vi "Autonomous Independent.vi"() -> ()   [LabVIEW 2017]
doc: "This VI is called when autonomous begins, and will automatically be terminated when autonomous ends. You can carry out timed or sensor driven robot movement independently without needing to return to the caller."
uses:
  <vilib>/Rock Robotics/WPI/ThirdParty/Phoenix-LabVIEW/Motor Controller/Controls/CTRE_Phoenix_MotorControl_ControlMode.ctl
  <vilib>/Rock Robotics/WPI/ThirdParty/Phoenix-LabVIEW/Pigeon IMU/CTRE_PigeonIMU_TareType.ctl
  Robot Global Data.vi
  <vilib>/Rock Robotics/Network Tables/NT Read Number.vi
panel:
  in  "Kp 4":dbl=0.015
  in  "Speed Dr str 4":dbl=1.0
  out "dis 3":i32
  out "Right Pos 2":i32
  in  "Kp 3":dbl=0.012
  in  "Speed Dr str 3":dbl=-0.5
  in  "Kp":dbl=0.015
  in  "Speed Dr str":dbl=1.0
  out "dis 2":i32
  out "Right Pos":i32
  in  "Kp 8":dbl=0.015
  in  "Speed Dr str 8":dbl=-1.0
  out "dis 7":i32
  out "Right Pos 6":i32
  in  "Kp 7":dbl=0.015
  in  "Speed Dr str 7":dbl=-1.0
  out "dis 6":i32
  out "Right Pos 5":i32
  in  "Kp 6":dbl=0.015
  in  "Speed Dr str 6":dbl=1.0
  out "dis 5":i32
  out "Right Pos 4":i32
  in  "Kp 5":dbl=0.015
  in  "Speed Dr str 5":dbl=-0.75
  in  "Kp 2":dbl=0.015
  in  "Speed Dr str 2":dbl=1.0
  out "dis 4":i32
  out "Right Pos 3":i32
  in  "First move (ms) 2":i32=60
  in  "First move Right 2":dbl=-0.75
  in  "First Move Left 2":dbl=-0.75
  # "Be sure to right-click and choose Data Operations>>Make Current Value default if you want to save the array values with the VI"
  # "115in from wall to swicth"
  # "SWITCH"
  # "SCALE"
  # "Correct"
  # "STRAIGHT SWITCH"
  # "-220"
  # "L"
  # "Staright auto"
  # ".117"
  # ".0041"
  # "=========================================================="
  # "Not correct"
  # "Get cube other side"
  # "R"
  # "other side"
  # "put 2nd cube in scale"
  # "find cube"
  # "waypt drive"
  # "Switch(new) Left"
  # "Switch(new) Right"
types:
  T1 = enum16{"FollowerType_PercentOutput", "FollowerType_AuxOutput1"}
  T2 = typedef "CTRE_PigeonIMU_TareType.ctl" = u8
  T3 = typedef "CTRE_Phoenix_MotorControl_ControlMode.ctl" = u16
  T4 = typedef "WPI_MotorControlDeviceRef.ctl" = cluster{"DeviceStatus":errorcluster, "Type":T5, "PWM":cluster{"PWM Channel":T6, "DeadBand":T7}, "CAN":cluster{"Device Number":u8, "SetOutput VI Ref":variant, "GetOutput VI Ref":variant, "Enable VI Ref":variant, "Disable VI Ref":variant, "Data":variant}, "Invert":bool, "DIO PWM":cluster{"PWM \"Enable\" Channel":T6, "DIOChannel":T8, "PWM Rate":dbl}}
  T5 = typedef "WPI_MotorControlType.ctl" = enum16{"PWM", "CAN", "DIO PWM"}
  T6 = typedef "FPGA_DIOPWMChannel.ctl" = enum8{"PWM 0", "PWM 1", "PWM 2", "PWM 3", "PWM 4", "PWM 5", "PWM 6", "PWM 7", "PWM 8", "PWM 9", "PWM MXP 0", "PWM MXP 1", "PWM MXP 2", "PWM MXP 3", "PWM MXP 4", "PWM MXP 5", "PWM MXP 6", "PWM MXP 7", "PWM MXP 8", "PWM MXP 9", "Invalid"}
  T7 = typedef "WPI_PWMDeadband.ctl" = cluster{"Name":string, "maxPositivePwm":i32, "minPositivePwm":i32, "centerPwm":i32, "maxNegativePwm":i32, "minNegativePwm":i32, "angularRange":u16}
  T8 = typedef "FPGA_DIOChannel.ctl" = enum8{"DIO 0", "DIO 1", "DIO 2", "DIO 3", "DIO 4", "DIO 5", "DIO 6", "DIO 7", "DIO 8", "DIO 9", "DIO MXP 0", "DIO MXP 1", "DIO MXP 2", "DIO MXP 3", "DIO MXP 4", "DIO MXP 5", "DIO MXP 6", "DIO MXP 7", "DIO MXP 8", "DIO MXP 9", "DIO MXP 10", "DIO MXP 11", "DIO MXP 12", "DIO MXP 13", "DIO MXP 14", "DIO MXP 15", "SPI Port CS1", "SPI Port CS2", "SPI Port CS3", "SPI Port MISO", "SPI Port MOSI", "Invalid"}
  T9 = typedef "CTRE_PigeonIMU_DeviceRef.ctl" = cluster{"DeviceStatus":errorcluster, "Device Number":u8, "Type":T10, "Device ID":u32, "Handle":u64, "UsageFrame":u32, "Library Path":path}
  T10 = typedef "CTRE_PigeonIMU_ConnectionType.ctl" = u32
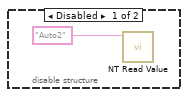
[diagram p2: hidden frame]
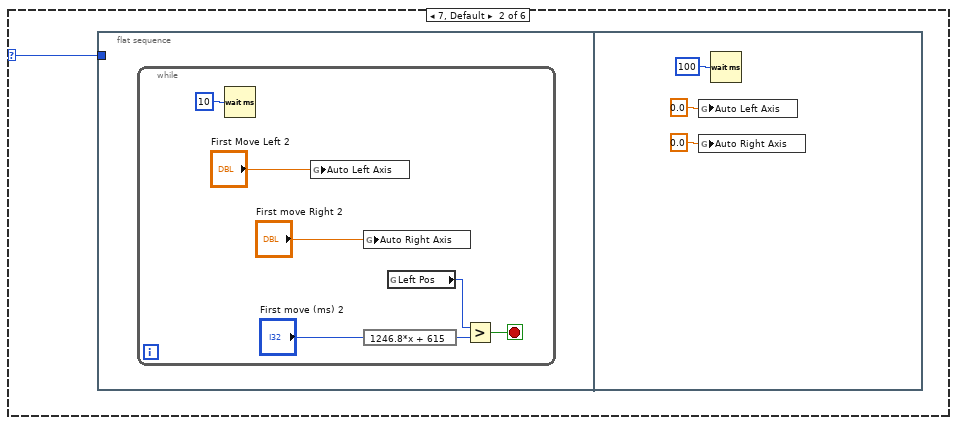
[diagram p3: hidden frame]
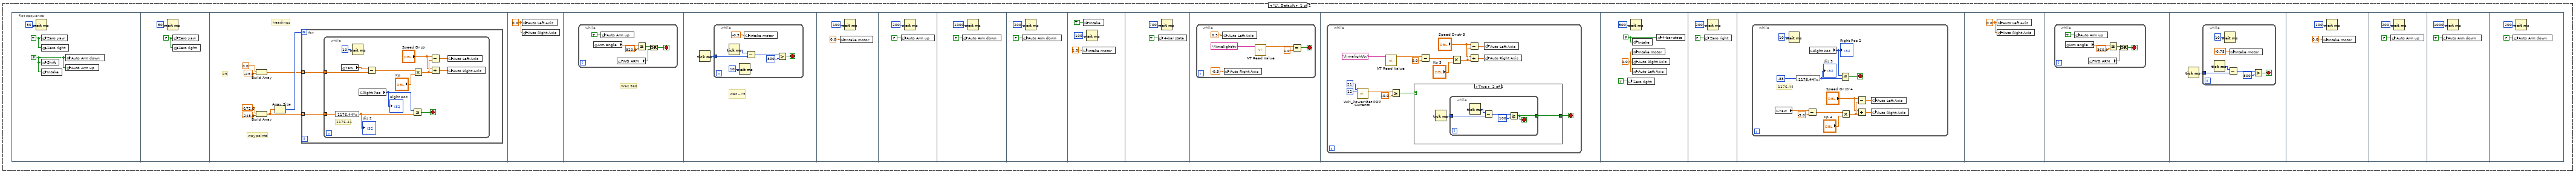
[diagram p5: hidden frame]
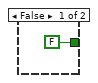
[diagram p6: hidden frame]
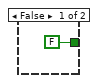
[diagram p7: hidden frame]
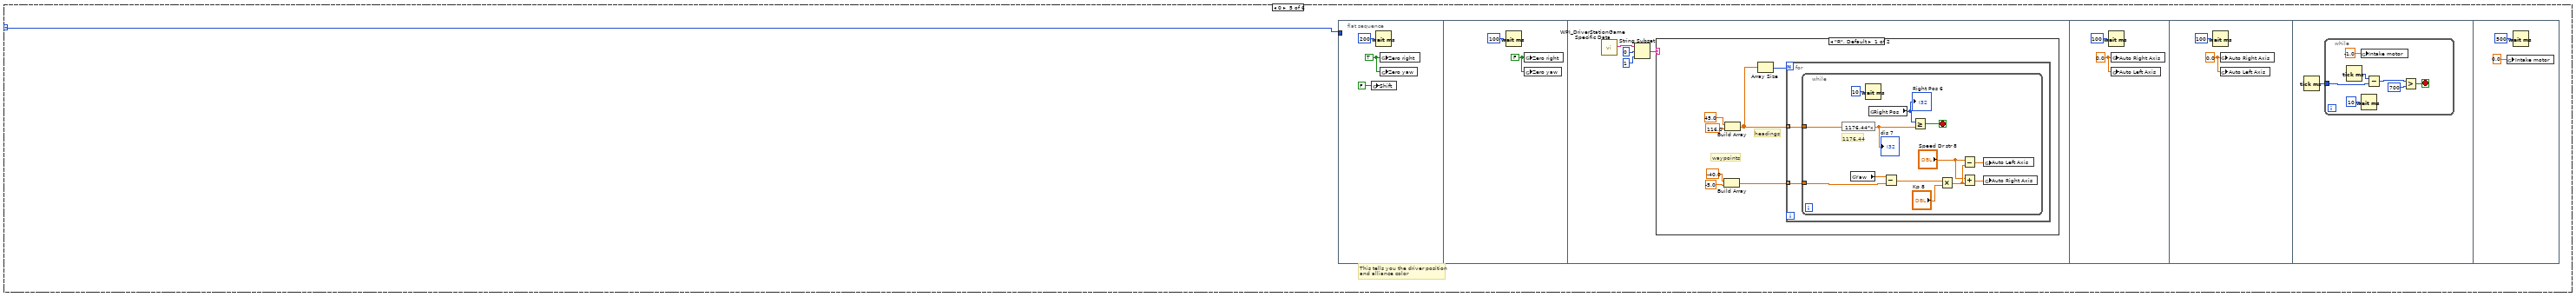
[diagram p9: hidden frame]
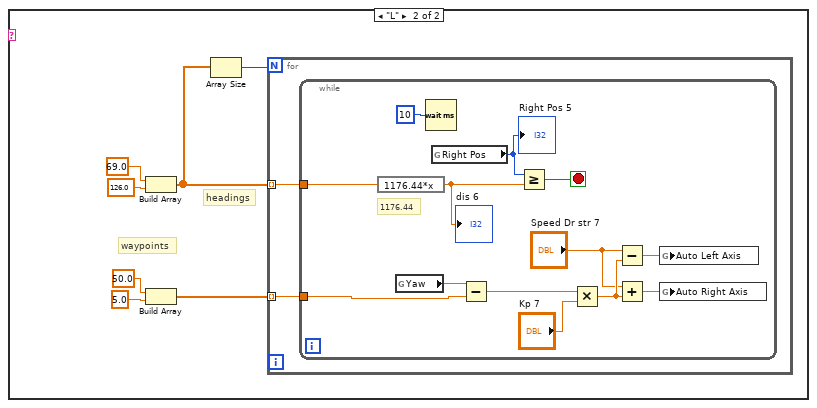
[diagram p10: hidden frame]
diagram:
  (unwired) "This function is run in parallel when the autonomous period begins. It will be terminated automatically when the period ends.\n\nNote that all Driver Station inputs are automatically latched and will not change once auto begins."
  # "Use time and/or sensors to control how the robot drives."
  # "Every 20ms, report that we are running autonomous\ncode. Loop will abort the same time as the VI."
  n1 = disable-structure shown="Enabled" {
    frame Disabled {
      n2 = call-poly <vilib>:"NT Read Value.vi"("Name"="Auto2") -> ()  [unwired: 9 in, 2 out]
    }
    frame Enabled {
    }
  }
  n3 = while {
    stop <- FALSE stop-if-true
    n4 = call <vilib>:"WPI_DriverStationReport Robot Code State.vi"("Autonomous"=TRUE) -> ()  [unwired: 10 in, 1 out]
    n5 = Wait (ms)(milliseconds to wait=u32 20) -> ()  [unwired: 1 out]
  }
  n6 = case shown="9" 9 {
    selector: 9 -> [_ w42 _ _ w336 _]
    frame 9 {
      w16 = T2 0 items=["SetValue"=0, "AddOffset"=1, "MatchCompass"=2, "SetOffset"=255] ("TareType (SetValue)")
      w6 = 0 ("New Sensor Position")
      w28 = 0.0 ("Output")
      w29 = T3 10 items=["PercentOutput"=0, "Position"=1, "Velocity"=2, "Current"=3, "Follower"=5, "MotionProfile"=6, "MotionMagic"=7, "MotionMagicArc"=8, "MotionProfileArc"=10, "Disabled"=15] ("Control Mode")
      w31 = T3 10 items=["PercentOutput"=0, "Position"=1, "Velocity"=2, "Current"=3, "Follower"=5, "MotionProfile"=6, "MotionMagic"=7, "MotionMagicArc"=8, "MotionProfileArc"=10, "Disabled"=15] ("Control Mode")
      n7 = call <vilib>:"CTRE_Phoenix_MotorControl_RefNumRegistryGet.vi"("refnum name"="Left encode") -> ("error out"=w26:errorcluster, "PhoenixMotorControlDevRef"=w24:T4)  [unwired: 9 in]
      n8 = call <vilib>:"CTRE_Phoenix_MotorControl_RefNumRegistryGet.vi"("refnum name"="Right encode") -> ("error out"=w27:errorcluster, "PhoenixMotorControlDevRef"=w23:T4)  [unwired: 9 in]
      n9 = call <vilib>:"CTRE_Phoenix_MotorControl_Set.vi"("error in (no error)"=w26, "Output"=w28, "Control Mode"=w29, "PhoenixMotorControlDevRef"=w24) -> ("error out"=w11:errorcluster, "PhoenixMotorControlDevRef"=w12:T4)  [unwired: 6 in]
      n10 = call <vilib>:"CTRE_Phoenix_MotorControl_Set.vi"("error in (no error)"=w27, "Output"=w28, "Control Mode"=w29, "PhoenixMotorControlDevRef"=w23) -> ("error out"=w7:errorcluster, "PhoenixMotorControlDevRef"=w10:T4)  [unwired: 6 in]
      n11 = call <vilib>:"CTRE_PigeonIMU_RefNumRegistryGet.vi"("refnum name"="imu") -> ("error out"=w14:errorcluster, "PigeonIMUDevRef"=w19:T9)  [unwired: 9 in]
      n12 = call <vilib>:"CTRE_Phoenix_MotorControl_SetQuadraturePosition_Enhanced.vi"("error in (no error)"=w11, "New Position"=w6, "PhoenixMotorControlDevRef"=w12) -> ("PhoenixMotorControlDevRef"=w13:T4)  [unwired: 7 in, 1 out]
      n13 = call <vilib>:"CTRE_Phoenix_MotorControl_SetQuadraturePosition_Enhanced.vi"("error in (no error)"=w7, "New Position"=w6, "PhoenixMotorControlDevRef"=w10) -> ("error out"=w8:errorcluster, "PhoenixMotorControlDevRef"=w9:T4)  [unwired: 7 in]
      n14 = call <vilib>:"CTRE_PigeonIMU_SetYaw.vi"("error in (no error)"=w14, "TareType (SetValue)"=w16, "Value"=0.0, "PigeonIMUDevRef"=w19) -> ()  [unwired: 6 in, 2 out]
      n15 = call <vilib>:"CTRE_Phoenix_MotorControl_ClearMotionProfileTrajectories.vi"("PhoenixMotorControlDevRef"=w9, "error in"=w8) -> ("PhoenixMotorControlDevRef"=w22:T4)  [unwired: 12 in, 1 out]
      n16 = call "Load Motion Profile.vi"("file path (dialog if empty)"=path "/home/lvuser/trajectories/right_cross.csv", "Right_Talon"=w22) -> ()  [unwired: 10 in]
      n17 = while {
        tunnel: [w39] -> w21
        tunnel: w13 -> [w39]
        tunnel: [w38] -> w15
        tunnel: w22 -> [w38]
        stop <- w41 stop-if-true
        n18 = global read "Robot Global Data.vi" "MP Cursor"() -> (w37:i32)
        n19 = Greater Or Equal?(x=w37, y=5) -> (x >= y?=w41:bool)
      }
      n20 = call <vilib>:"CTRE_Phoenix_MotorControl_Set.vi"("Output"=1.0, "Control Mode"=w31, "PhoenixMotorControlDevRef"=w15) -> ()  [unwired: 7 in, 2 out]
      n21 = call <vilib>:"CTRE_Phoenix_MotorControl_Follow.vi"("FollowerType"=T1."FollowerType_AuxOutput1", "Master Controller to Follow"=w15, "PhoenixMotorControlDevRef"=w21) -> ()  [unwired: 7 in, 2 out]
      n22 = while {
        tunnel: w15 -> [w36]
        stop <- FALSE stop-if-true
        n23 = call <vilib>:"CTRE_Phoenix_MotorControl_ProcessMotionProfileBuffer.vi"("PhoenixMotorControlDevRef"=w36) -> ()  [unwired: 13 in, 2 out]
        n24 = Wait (ms)(milliseconds to wait=u32 5) -> ()  [unwired: 1 out]
      }
    }
    frame 7, Default {
      n25 = flat-sequence {
        tunnel: w42 -> [_]
        frame #0 {
          n26 = while {
            stop <- w49 stop-if-true
            n27 = Wait (ms)(milliseconds to wait=u32 10) -> ()  [unwired: 1 out]
            n28 = global write "Robot Global Data.vi" "Auto Left Axis"("First Move Left 2") -> ()
            n29 = global write "Robot Global Data.vi" "Auto Right Axis"("First move Right 2") -> ()
            n30 = expression code="1246.8*x + 615"("First move (ms) 2") -> (w44:i32)
            n31 = global read "Robot Global Data.vi" "Left Pos"() -> (w43:i32)
            n32 = Greater?(x=w43, y=w44) -> (0:w49:bool)
          }
        }
        frame #1 {
          n33 = global write "Robot Global Data.vi" "Auto Left Axis"(0.0 ("Auto Left Axis")) -> ()
          n34 = global write "Robot Global Data.vi" "Auto Right Axis"(0.0 ("Auto Left Axis")) -> ()
          n35 = Wait (ms)(milliseconds to wait=u32 100) -> ()  [unwired: 1 out]
        }
      }
    }
    frame 3 {
      n36 = call <vilib>:"WPI_DriverStationGame Specific Data.vi"() -> ("Game Specific Data"=w56:string)  [unwired: 11 in]
      n37 = String Subset(string=w56, offset (0)=1, length (rest)=1 ("length (rest)")) -> (substring=w53:string)
      n38 = case shown="\"R\"" w53 {
        frame "L", Default {
          n39 = flat-sequence {
            frame #0 {
              w57 = FALSE
              w58 = TRUE ("Zero right")
              n40 = Wait (ms)(milliseconds to wait=u32 50) -> ()  [unwired: 1 out]
              n41 = global write "Robot Global Data.vi" "Zero yaw"(w58) -> ()
              n42 = global write "Robot Global Data.vi" "Zero right"(w58) -> ()
              n43 = global write "Robot Global Data.vi" "Shift"(w57) -> ()
              n44 = global write "Robot Global Data.vi" "Intake"(w57) -> ()
              n45 = global write "Robot Global Data.vi" "Auto Arm down"(w57) -> ()
              n46 = global write "Robot Global Data.vi" "Auto Arm up"(w57) -> ()
            }
            frame #1 {
              w60 = FALSE ("Zero right")
              n47 = Wait (ms)(milliseconds to wait=u32 50) -> ()  [unwired: 1 out]
              n48 = global write "Robot Global Data.vi" "Zero yaw"(w60) -> ()
              n49 = global write "Robot Global Data.vi" "Zero right"(w60) -> ()
            }
            frame #2 {
              # "25"
              # "waypoints"
              # "headings"
              n50 = Build Array(0.0 ("element"), -23.0 ("element")) -> (w62:dbl[])
              n51 = Build Array(-172.0 ("element"), -248.0 ("element")) -> (w63:dbl[])
              n52 = Array Size(array=w63) -> (size(s)=w68:i32)
              n53 = for {
                N: w68 -> [_]
                tunnel: w63 -> [w70] mode=indexing
                tunnel: w62 -> [w69] mode=indexing
                n54 = while {
                  tunnel: w70 -> [w75]
                  tunnel: w69 -> [w71]
                  stop <- w80 stop-if-true
                  # "1176.44"
                  n55 = expression code="1176.44*x"(w75) -> (w76:dbl)
                  "dis 2" <- w76
                  n56 = global read "Robot Global Data.vi" "Yaw"() -> (w72:dbl)
                  n57 = Wait (ms)(milliseconds to wait=u32 10) -> ()  [unwired: 1 out]
                  n58 = global read "Robot Global Data.vi" "Right Pos"() -> (w73:i32)
                  "Right Pos" <- w73
                  n59 = Subtract(x=w72, y=w71) -> (x-y=w74:dbl)
                  n60 = Less Or Equal?(x=w73, y=w76) -> (x <= y?=w80:bool)
                  n61 = Multiply(x=w74, y="Kp") -> (x*y=w79:dbl)
                  n62 = Subtract(x="Speed Dr str", y=w79) -> (x-y=w82:dbl)
                  n63 = Add(x="Speed Dr str", y=w79) -> (x+y=w81:dbl)
                  n64 = global write "Robot Global Data.vi" "Auto Left Axis"(w82) -> ()
                  n65 = global write "Robot Global Data.vi" "Auto Right Axis"(w81) -> ()
                }
              }
            }
            frame #3 {
              w84 = 0.0
              n66 = global write "Robot Global Data.vi" "Auto Left Axis"(w84) -> ()
              n67 = global write "Robot Global Data.vi" "Auto Right Axis"(w84) -> ()
            }
            frame #4 {
              # "Was 360"
              n68 = while {
                stop <- w85 stop-if-true
                n69 = global read "Robot Global Data.vi" "Arm angle"() -> (w89:dbl)
                n70 = global write "Robot Global Data.vi" "Auto Arm up"(TRUE) -> ()
                n71 = global read "Robot Global Data.vi" "FWD ARM"() -> (w86:bool)
                n72 = Greater Or Equal?(x=w89, y=320.0) -> (x >= y?=w87:bool)
                n73 = Or(x=w87, y=w86) -> (x .or. y?=w85:bool)
              }
            }
            frame #5 {
              # "was -.75"
              n74 = Tick Count (ms)() -> (millisecond timer value=w91:u32)
              n75 = while {
                tunnel: w91 -> [w96]
                stop <- w93 stop-if-true
                n76 = Tick Count (ms)() -> (millisecond timer value=w97:u32)
                n77 = Wait (ms)(milliseconds to wait=u32 10) -> ()  [unwired: 1 out]
                n78 = global write "Robot Global Data.vi" "Intake motor"(-0.5 ("Intake motor")) -> ()
                n79 = Subtract(x=w97, y=w96) -> (x-y=w95:u32)
                n80 = Greater?(x=w95, y=u32 800) -> (0:w93:bool)
              }
            }
            frame #6 {
              n81 = global write "Robot Global Data.vi" "Intake motor"(0.0 ("Intake motor")) -> ()
              n82 = Wait (ms)(milliseconds to wait=u32 100) -> ()  [unwired: 1 out]
            }
            frame #7 {
              n83 = global write "Robot Global Data.vi" "Auto Arm up"(FALSE) -> ()
              n84 = Wait (ms)(milliseconds to wait=u32 200) -> ()  [unwired: 1 out]
            }
            frame #8 {
              n85 = global write "Robot Global Data.vi" "Auto Arm down"(TRUE) -> ()
              n86 = Wait (ms)(milliseconds to wait=u32 1000) -> ()  [unwired: 1 out]
            }
            frame #9 {
              n87 = global write "Robot Global Data.vi" "Auto Arm down"(FALSE) -> ()
              n88 = Wait (ms)(milliseconds to wait=u32 200) -> ()  [unwired: 1 out]
            }
            frame #10 {
              n89 = global write "Robot Global Data.vi" "Intake motor"(1.0 ("Intake motor")) -> ()
              n90 = global write "Robot Global Data.vi" "Intake"(TRUE ("Intake")) -> ()
              n91 = Wait (ms)(milliseconds to wait=u32 100) -> ()  [unwired: 1 out]
            }
            frame #11 {
              n92 = global write "Robot Global Data.vi" "4-bar state"(TRUE ("4-bar state")) -> ()
              n93 = Wait (ms)(milliseconds to wait=u32 700) -> ()  [unwired: 1 out]
            }
            frame #12 {
              n94 = while {
                stop <- w112 stop-if-true
                n95 = global write "Robot Global Data.vi" "Auto Left Axis"(0.5 ("Auto Left Axis")) -> ()
                n96 = global write "Robot Global Data.vi" "Auto Right Axis"(-0.5 ("Auto Right Axis")) -> ()
                n97 = call-poly <vilib>:"NT Read Value.vi"("Name"="/limelight/tv") -> ("Numeric"=w114:dbl)  [unwired: 9 in, 1 out]
                n98 = Equal?(x=w114, y=1.0) -> (x = y?=w112:bool)
              }
            }
            frame #13 {
              n99 = while {
                stop <- w132 stop-if-true
                n100 = call <vilib>:"WPI_Power Get PDP Currents.vi"("Power Distribution Panel (0)"=u8 21, "PDP Channel"=12) -> ("current (A)"=w127:dbl)  [unwired: 11 in, 2 out]
                n101 = call-poly <vilib>:"NT Read Value.vi"("Name"="/limelight/tx") -> ("Numeric"=w119:dbl)  [unwired: 9 in, 1 out]
                n102 = Greater Or Equal?(x=w127, y=40.0 ("x")) -> (x >= y?=w129:bool)
                n103 = case shown="True" w129 {
                  tunnel: [FALSE w134] -> w132
                  frame False {
                  }
                  frame True {
                    n104 = Tick Count (ms)() -> (millisecond timer value=w135:u32)
                    n105 = while {
                      tunnel: w135 -> [w139]
                      tunnel: [w136] -> w134
                      stop <- w136 stop-if-true
                      n106 = Tick Count (ms)() -> (millisecond timer value=w140:u32)
                      n107 = Subtract(x=w140, y=w139) -> (x-y=w138:u32)
                      n108 = Greater Or Equal?(x=w138, y=u32 100) -> (x >= y?=w136:bool)
                    }
                  }
                }
                n109 = Subtract(x=w119, y=0.0) -> (x-y=w121:dbl)
                n110 = Multiply(x=w121, y="Kp 3") -> (x*y=w123:dbl)
                n111 = Subtract(x="Speed Dr str 3", y=w123) -> (x-y=w125:dbl)
                n112 = Add(x="Speed Dr str 3", y=w123) -> (x+y=w124:dbl)
                n113 = global write "Robot Global Data.vi" "Auto Left Axis"(w125) -> ()
                n114 = global write "Robot Global Data.vi" "Auto Right Axis"(w124) -> ()
              }
            }
            frame #14 {
              w141 = FALSE ("4-bar state")
              w144 = 0.0 ("Intake motor")
              n115 = global write "Robot Global Data.vi" "Zero right"(TRUE) -> ()
              n116 = Wait (ms)(milliseconds to wait=u32 500) -> ()  [unwired: 1 out]
              n117 = global write "Robot Global Data.vi" "Intake"(w141) -> ()
              n118 = global write "Robot Global Data.vi" "Intake motor"(w144) -> ()
              n119 = global write "Robot Global Data.vi" "Auto Right Axis"(w144) -> ()
              n120 = global write "Robot Global Data.vi" "Auto Left Axis"(w144) -> ()
              n121 = global write "Robot Global Data.vi" "4-bar state"(w141) -> ()
            }
            frame #15 {
              n122 = global write "Robot Global Data.vi" "Zero right"(FALSE) -> ()
              n123 = Wait (ms)(milliseconds to wait=u32 200) -> ()  [unwired: 1 out]
            }
            frame #16 {
              n124 = while {
                stop <- w156 stop-if-true
                # "1176.44"
                n125 = global read "Robot Global Data.vi" "Yaw"() -> (w150:dbl)
                n126 = Wait (ms)(milliseconds to wait=u32 10) -> ()  [unwired: 1 out]
                n127 = expression code="1176.44*x"(-35) -> (w152:i32)
                "dis 3" <- w152
                n128 = Subtract(x=w150, y=-5.0) -> (x-y=w151:dbl)
                n129 = global read "Robot Global Data.vi" "Right Pos"() -> (w149:i32)
                "Right Pos 2" <- w149
                n130 = Less Or Equal?(x=w149, y=w152) -> (x <= y?=w156:bool)
                n131 = Multiply(x=w151, y="Kp 4") -> (x*y=w155:dbl)
                n132 = Subtract(x="Speed Dr str 4", y=w155) -> (x-y=w158:dbl)
                n133 = Add(x="Speed Dr str 4", y=w155) -> (x+y=w157:dbl)
                n134 = global write "Robot Global Data.vi" "Auto Left Axis"(w158) -> ()
                n135 = global write "Robot Global Data.vi" "Auto Right Axis"(w157) -> ()
              }
            }
            frame #17 {
              w160 = 0.0
              n136 = global write "Robot Global Data.vi" "Auto Left Axis"(w160) -> ()
              n137 = global write "Robot Global Data.vi" "Auto Right Axis"(w160) -> ()
            }
            frame #18 {
              n138 = while {
                stop <- w161 stop-if-true
                n139 = global read "Robot Global Data.vi" "Arm angle"() -> (w165:dbl)
                n140 = global write "Robot Global Data.vi" "Auto Arm up"(TRUE) -> ()
                n141 = global read "Robot Global Data.vi" "FWD ARM"() -> (w162:bool)
                n142 = Greater Or Equal?(x=w165, y=360.0) -> (x >= y?=w163:bool)
                n143 = Or(x=w163, y=w162) -> (x .or. y?=w161:bool)
              }
            }
            frame #19 {
              n144 = Tick Count (ms)() -> (millisecond timer value=w167:u32)
              n145 = while {
                tunnel: w167 -> [w172]
                stop <- w169 stop-if-true
                n146 = Tick Count (ms)() -> (millisecond timer value=w173:u32)
                n147 = Wait (ms)(milliseconds to wait=u32 10) -> ()  [unwired: 1 out]
                n148 = Subtract(x=w173, y=w172) -> (x-y=w171:u32)
                n149 = global write "Robot Global Data.vi" "Intake motor"(-0.75 ("Intake motor")) -> ()
                n150 = Greater?(x=w171, y=u32 800) -> (0:w169:bool)
              }
            }
            frame #20 {
              n151 = global write "Robot Global Data.vi" "Intake motor"(0.0 ("Intake motor")) -> ()
              n152 = Wait (ms)(milliseconds to wait=u32 100) -> ()  [unwired: 1 out]
            }
            frame #21 {
              n153 = global write "Robot Global Data.vi" "Auto Arm up"(FALSE) -> ()
              n154 = Wait (ms)(milliseconds to wait=u32 200) -> ()  [unwired: 1 out]
            }
            frame #22 {
              n155 = global write "Robot Global Data.vi" "Auto Arm down"(TRUE) -> ()
              n156 = Wait (ms)(milliseconds to wait=u32 1000) -> ()  [unwired: 1 out]
            }
            frame #23 {
              n157 = global write "Robot Global Data.vi" "Auto Arm down"(FALSE) -> ()
              n158 = Wait (ms)(milliseconds to wait=u32 200) -> ()  [unwired: 1 out]
            }
          }
        }
        frame "R" {
          # "other side"
          n159 = flat-sequence {
            frame #0 {
              w187 = TRUE ("4-bar state")
              n160 = global write "Robot Global Data.vi" "Auto Right Axis"(0.0 ("Auto Right Axis")) -> ()
              n161 = global write "Robot Global Data.vi" "Auto Left Axis"(0.0 ("Auto Left Axis")) -> ()
              n162 = global write "Robot Global Data.vi" "4-bar state"(FALSE ("4-bar state")) -> ()
              n163 = Wait (ms)(milliseconds to wait=u32 50) -> ()  [unwired: 1 out]
              n164 = global write "Robot Global Data.vi" "Zero right"(w187) -> ()
              n165 = global write "Robot Global Data.vi" "Zero yaw"(w187) -> ()
            }
            frame #1 {
              w189 = FALSE ("4-bar state")
              n166 = Wait (ms)(milliseconds to wait=u32 50) -> ()  [unwired: 1 out]
              n167 = global write "Robot Global Data.vi" "Zero right"(w189) -> ()
              n168 = global write "Robot Global Data.vi" "Zero yaw"(w189) -> ()
            }
            frame #2 {
              # "-237"
              # "-400"
              # "waypoints"
              # "headings"
              n169 = Build Array(-170.0 ("element"), -200.0 ("element"), -237.0 ("element"), -400.0 ("element")) -> (w195:dbl[])
              n170 = Array Size(array=w195) -> (size(s)=w200:i32)
              n171 = Build Array(0.0 ("element"), -30.0 ("element"), -90.0 ("element"), -90.0 ("element")) -> (w194:dbl[])
              n172 = for {
                N: w200 -> [_]
                tunnel: w195 -> [w202] mode=indexing
                tunnel: w194 -> [w201] mode=indexing
                n173 = while {
                  tunnel: w202 -> [w207]
                  tunnel: w201 -> [w203]
                  stop <- w212 stop-if-true
                  # "1176.44"
                  n174 = expression code="1176.44*x"(w207) -> (w208:dbl)
                  "dis 4" <- w208
                  n175 = global read "Robot Global Data.vi" "Yaw"() -> (w204:dbl)
                  n176 = Wait (ms)(milliseconds to wait=u32 10) -> ()  [unwired: 1 out]
                  n177 = global read "Robot Global Data.vi" "Right Pos"() -> (w205:i32)
                  "Right Pos 3" <- w205
                  n178 = Subtract(x=w204, y=w203) -> (x-y=w206:dbl)
                  n179 = Less Or Equal?(x=w205, y=w208) -> (x <= y?=w212:bool)
                  n180 = Multiply(x=w206, y="Kp 2") -> (x*y=w211:dbl)
                  n181 = Subtract(x="Speed Dr str 2", y=w211) -> (x-y=w214:dbl)
                  n182 = Add(x="Speed Dr str 2", y=w211) -> (x+y=w213:dbl)
                  n183 = global write "Robot Global Data.vi" "Auto Left Axis"(w214) -> ()
                  n184 = global write "Robot Global Data.vi" "Auto Right Axis"(w213) -> ()
                }
              }
            }
            frame #3 {
              w216 = 0.0
              n185 = global write "Robot Global Data.vi" "Auto Left Axis"(w216) -> ()
              n186 = global write "Robot Global Data.vi" "Auto Right Axis"(w216) -> ()
            }
            frame #4 {
              n187 = while {
                stop <- w218 stop-if-true
                n188 = global read "Robot Global Data.vi" "Yaw"() -> (w220:dbl)
                n189 = Wait (ms)(milliseconds to wait=u32 10) -> ()  [unwired: 1 out]
                n190 = global write "Robot Global Data.vi" "Auto Left Axis"(0.75) -> ()
                n191 = global write "Robot Global Data.vi" "Auto Right Axis"(-0.75) -> ()
                n192 = Greater Or Equal?(x=w220, y=-15.0) -> (x >= y?=w218:bool)
              }
            }
            frame #5 {
              w224 = 0.0
              n193 = Wait (ms)(milliseconds to wait=u32 20) -> ()  [unwired: 1 out]
              n194 = global write "Robot Global Data.vi" "Auto Left Axis"(w224) -> ()
              n195 = global write "Robot Global Data.vi" "Auto Right Axis"(w224) -> ()
            }
            frame #6 {
              n196 = global write "Robot Global Data.vi" "Zero right"(TRUE ("Zero right")) -> ()
              n197 = Wait (ms)(milliseconds to wait=u32 150) -> ()  [unwired: 1 out]
            }
            frame #7 {
              n198 = global write "Robot Global Data.vi" "Zero right"(FALSE ("Zero right")) -> ()
              n199 = Wait (ms)(milliseconds to wait=u32 50) -> ()  [unwired: 1 out]
            }
            frame #8 {
              n200 = while {
                stop <- w230 stop-if-true
                w234 = 1.0
                n201 = Wait (ms)(milliseconds to wait=u32 10) -> ()  [unwired: 1 out]
                n202 = global write "Robot Global Data.vi" "Auto Left Axis"(w234) -> ()
                n203 = global write "Robot Global Data.vi" "Auto Right Axis"(w234) -> ()
                n204 = global read "Robot Global Data.vi" "Right Pos"() -> (w233:i32)
                n205 = expression code="1176.44*x"(-12.0 ("element")) -> (w232:dbl)
                n206 = Less Or Equal?(x=w233, y=w232) -> (x <= y?=w230:bool)
              }
            }
            frame #9 {
              w236 = 0.0
              n207 = Wait (ms)(milliseconds to wait=u32 20) -> ()  [unwired: 1 out]
              n208 = global write "Robot Global Data.vi" "Auto Left Axis"(w236) -> ()
              n209 = global write "Robot Global Data.vi" "Auto Right Axis"(w236) -> ()
            }
            frame #10 {
              # "was 300"
              n210 = while {
                stop <- w237 stop-if-true
                n211 = global read "Robot Global Data.vi" "Arm angle"() -> (w241:dbl)
                n212 = global write "Robot Global Data.vi" "Auto Arm up"(TRUE) -> ()
                n213 = global read "Robot Global Data.vi" "FWD ARM"() -> (w238:bool)
                n214 = Greater Or Equal?(x=w241, y=290.0) -> (x >= y?=w239:bool)
                n215 = Or(x=w239, y=w238) -> (x .or. y?=w237:bool)
              }
            }
            frame #11 {
              # "was -.5"
              n216 = Tick Count (ms)() -> (millisecond timer value=w243:u32)
              n217 = while {
                tunnel: w243 -> [w248]
                stop <- w245 stop-if-true
                n218 = Tick Count (ms)() -> (millisecond timer value=w249:u32)
                n219 = Wait (ms)(milliseconds to wait=u32 10) -> ()  [unwired: 1 out]
                n220 = global write "Robot Global Data.vi" "Intake motor"(-0.5 ("Intake motor")) -> ()
                n221 = Subtract(x=w249, y=w248) -> (x-y=w247:u32)
                n222 = Greater?(x=w247, y=u32 500) -> (0:w245:bool)
              }
            }
            frame #12 {
              n223 = global write "Robot Global Data.vi" "Intake motor"(0.0 ("Intake motor")) -> ()
              n224 = Wait (ms)(milliseconds to wait=u32 50) -> ()  [unwired: 1 out]
            }
            frame #13 {
              n225 = global write "Robot Global Data.vi" "Auto Arm up"(FALSE) -> ()
              n226 = global write "Robot Global Data.vi" "Auto Arm down"(TRUE ("Auto Arm down")) -> ()
              n227 = Wait (ms)(milliseconds to wait=u32 1000) -> ()  [unwired: 1 out]
            }
            frame #14 {
              n228 = global write "Robot Global Data.vi" "Auto Arm down"(FALSE) -> ()
              n229 = Wait (ms)(milliseconds to wait=u32 50) -> ()  [unwired: 1 out]
            }
            frame #15 {
              n230 = global write "Robot Global Data.vi" "Intake motor"(1.0 ("Intake motor")) -> ()
              n231 = global write "Robot Global Data.vi" "Intake"(TRUE ("Intake")) -> ()
              n232 = Wait (ms)(milliseconds to wait=u32 50) -> ()  [unwired: 1 out]
            }
            frame #16 {
              n233 = global write "Robot Global Data.vi" "4-bar state"(TRUE ("4-bar state")) -> ()
              n234 = Wait (ms)(milliseconds to wait=u32 700) -> ()  [unwired: 1 out]
            }
            frame #17 {
              n235 = Tick Count (ms)() -> (millisecond timer value=w263:u32)
              n236 = while {
                tunnel: w263 -> [w267]
                stop <- w264 stop-if-true
                n237 = Tick Count (ms)() -> (millisecond timer value=w268:u32)
                n238 = global write "Robot Global Data.vi" "Auto Right Axis"(1.0) -> ()
                n239 = global write "Robot Global Data.vi" "Auto Left Axis"(-1.0) -> ()
                n240 = Subtract(x=w268, y=w267) -> (x-y=w266:u32)
                n241 = Greater Or Equal?(x=w266, y=u32 100) -> (x >= y?=w264:bool)
              }
            }
            frame #18 {
              n242 = while {
                stop <- w285 stop-if-true
                n243 = call <vilib>:"WPI_Power Get PDP Currents.vi"("Power Distribution Panel (0)"=u8 21, "PDP Channel"=12) -> ("current (A)"=w280:dbl)  [unwired: 11 in, 2 out]
                n244 = call-poly <vilib>:"NT Read Value.vi"("Name"="/limelight/tx") -> ("Numeric"=w272:dbl)  [unwired: 9 in, 1 out]
                n245 = Greater Or Equal?(x=w280, y=40.0 ("x")) -> (x >= y?=w282:bool)
                n246 = case shown="True" w282 {
                  tunnel: [FALSE w287] -> w285
                  frame False {
                  }
                  frame True {
                    n247 = Tick Count (ms)() -> (millisecond timer value=w288:u32)
                    n248 = while {
                      tunnel: w288 -> [w292]
                      tunnel: [w289] -> w287
                      stop <- w289 stop-if-true
                      n249 = Tick Count (ms)() -> (millisecond timer value=w293:u32)
                      n250 = Subtract(x=w293, y=w292) -> (x-y=w291:u32)
                      n251 = Greater Or Equal?(x=w291, y=u32 70) -> (x >= y?=w289:bool)
                    }
                  }
                }
                n252 = Subtract(x=w272, y=0.0) -> (x-y=w274:dbl)
                n253 = Multiply(x=w274, y="Kp 5") -> (x*y=w276:dbl)
                n254 = Subtract(x="Speed Dr str 5", y=w276) -> (x-y=w278:dbl)
                n255 = Add(x="Speed Dr str 5", y=w276) -> (x+y=w277:dbl)
                n256 = global write "Robot Global Data.vi" "Auto Left Axis"(w278) -> ()
                n257 = global write "Robot Global Data.vi" "Auto Right Axis"(w277) -> ()
              }
            }
            frame #19 {
              w294 = FALSE ("4-bar state")
              w297 = 0.0 ("Intake motor")
              n258 = global write "Robot Global Data.vi" "Zero right"(TRUE) -> ()
              n259 = Wait (ms)(milliseconds to wait=u32 150) -> ()  [unwired: 1 out]
              n260 = global write "Robot Global Data.vi" "Intake"(w294) -> ()
              n261 = global write "Robot Global Data.vi" "Intake motor"(w297) -> ()
              n262 = global write "Robot Global Data.vi" "Auto Right Axis"(w297) -> ()
              n263 = global write "Robot Global Data.vi" "Auto Left Axis"(w297) -> ()
              n264 = global write "Robot Global Data.vi" "4-bar state"(w294) -> ()
            }
            frame #20 {
              n265 = global write "Robot Global Data.vi" "Zero right"(FALSE) -> ()
              n266 = Wait (ms)(milliseconds to wait=u32 50) -> ()  [unwired: 1 out]
            }
            frame #21 {
              n267 = while {
                stop <- w309 stop-if-true
                # "1176.44"
                n268 = global read "Robot Global Data.vi" "Yaw"() -> (w303:dbl)
                n269 = Wait (ms)(milliseconds to wait=u32 10) -> ()  [unwired: 1 out]
                n270 = expression code="1176.44*x"(-20) -> (w305:i32)
                "dis 5" <- w305
                n271 = Subtract(x=w303, y=0.0) -> (x-y=w304:dbl)
                n272 = global read "Robot Global Data.vi" "Right Pos"() -> (w302:i32)
                "Right Pos 4" <- w302
                n273 = Less Or Equal?(x=w302, y=w305) -> (x <= y?=w309:bool)
                n274 = Multiply(x=w304, y="Kp 6") -> (x*y=w308:dbl)
                n275 = Subtract(x="Speed Dr str 6", y=w308) -> (x-y=w311:dbl)
                n276 = Add(x="Speed Dr str 6", y=w308) -> (x+y=w310:dbl)
                n277 = global write "Robot Global Data.vi" "Auto Left Axis"(w311) -> ()
                n278 = global write "Robot Global Data.vi" "Auto Right Axis"(w310) -> ()
              }
            }
            frame #22 {
              w313 = 0.0
              n279 = global write "Robot Global Data.vi" "Auto Left Axis"(w313) -> ()
              n280 = global write "Robot Global Data.vi" "Auto Right Axis"(w313) -> ()
            }
            frame #23 {
              n281 = while {
                stop <- w314 stop-if-true
                n282 = global read "Robot Global Data.vi" "Arm angle"() -> (w318:dbl)
                n283 = global write "Robot Global Data.vi" "Auto Arm up"(TRUE) -> ()
                n284 = global read "Robot Global Data.vi" "FWD ARM"() -> (w315:bool)
                n285 = Greater Or Equal?(x=w318, y=300.0) -> (x >= y?=w316:bool)
                n286 = Or(x=w316, y=w315) -> (x .or. y?=w314:bool)
              }
            }
            frame #24 {
              n287 = Tick Count (ms)() -> (millisecond timer value=w320:u32)
              n288 = while {
                tunnel: w320 -> [w325]
                stop <- w322 stop-if-true
                n289 = Tick Count (ms)() -> (millisecond timer value=w326:u32)
                n290 = Wait (ms)(milliseconds to wait=u32 10) -> ()  [unwired: 1 out]
                n291 = global write "Robot Global Data.vi" "Intake motor"(-0.3 ("Intake motor")) -> ()
                n292 = Subtract(x=w326, y=w325) -> (x-y=w324:u32)
                n293 = Greater?(x=w324, y=u32 800) -> (0:w322:bool)
              }
            }
            frame #25 {
              n294 = global write "Robot Global Data.vi" "Intake motor"(0.0 ("Intake motor")) -> ()
              n295 = Wait (ms)(milliseconds to wait=u32 50) -> ()  [unwired: 1 out]
            }
            frame #26 {
              n296 = global write "Robot Global Data.vi" "Auto Arm up"(FALSE) -> ()
              n297 = Wait (ms)(milliseconds to wait=u32 200) -> ()  [unwired: 1 out]
            }
            frame #27 {
              n298 = global write "Robot Global Data.vi" "Auto Arm down"(TRUE) -> ()
              n299 = Wait (ms)(milliseconds to wait=u32 1000) -> ()  [unwired: 1 out]
            }
            frame #28 {
              n300 = global write "Robot Global Data.vi" "Auto Arm down"(FALSE) -> ()
              n301 = Wait (ms)(milliseconds to wait=u32 50) -> ()  [unwired: 1 out]
            }
          }
        }
      }
    }
    frame 1 {
    }
    frame 0 {
      # "This tells you the driver position\nand alliance color"
      n302 = flat-sequence {
        tunnel: w336 -> [_]
        frame #0 {
          w338 = TRUE
          n303 = global write "Robot Global Data.vi" "Shift"(FALSE ("Shift")) -> ()
          n304 = Wait (ms)(milliseconds to wait=u32 200) -> ()  [unwired: 1 out]
          n305 = global write "Robot Global Data.vi" "Zero right"(w338) -> ()
          n306 = global write "Robot Global Data.vi" "Zero yaw"(w338) -> ()
        }
        frame #1 {
          w340 = FALSE
          n307 = Wait (ms)(milliseconds to wait=u32 100) -> ()  [unwired: 1 out]
          n308 = global write "Robot Global Data.vi" "Zero right"(w340) -> ()
          n309 = global write "Robot Global Data.vi" "Zero yaw"(w340) -> ()
        }
        frame #2 {
          n310 = call <vilib>:"WPI_DriverStationGame Specific Data.vi"() -> ("Game Specific Data"=w345:string)  [unwired: 11 in]
          n311 = String Subset(string=w345, offset (0)=0, length (rest)=1 ("length (rest)")) -> (substring=w342:string)
          n312 = case shown="\"R\", Default" w342 {
            frame "R", Default {
              # "waypoints"
              # "headings"
              n313 = Build Array(-40.0 ("element"), -5.0 ("element")) -> (w352:dbl[])
              n314 = Build Array(45.0 ("element"), 116.0 ("element")) -> (w351:dbl[])
              n315 = Array Size(array=w351) -> (size(s)=w350:i32)
              n316 = for {
                N: w350 -> [_]
                tunnel: w351 -> [w354] mode=indexing
                tunnel: w352 -> [w353] mode=indexing
                n317 = while {
                  tunnel: w354 -> [w359]
                  tunnel: w353 -> [w355]
                  stop <- w364 stop-if-true
                  # "1176.44"
                  n318 = expression code="1176.44*x"(w359) -> (w360:dbl)
                  "dis 7" <- w360
                  n319 = global read "Robot Global Data.vi" "Yaw"() -> (w356:dbl)
                  n320 = Wait (ms)(milliseconds to wait=u32 10) -> ()  [unwired: 1 out]
                  n321 = global read "Robot Global Data.vi" "Right Pos"() -> (w357:i32)
                  "Right Pos 6" <- w357
                  n322 = Subtract(x=w356, y=w355) -> (x-y=w358:dbl)
                  n323 = Greater Or Equal?(x=w357, y=w360) -> (x >= y?=w364:bool)
                  n324 = Multiply(x=w358, y="Kp 8") -> (x*y=w363:dbl)
                  n325 = Subtract(x="Speed Dr str 8", y=w363) -> (x-y=w366:dbl)
                  n326 = Add(x="Speed Dr str 8", y=w363) -> (x+y=w365:dbl)
                  n327 = global write "Robot Global Data.vi" "Auto Left Axis"(w366) -> ()
                  n328 = global write "Robot Global Data.vi" "Auto Right Axis"(w365) -> ()
                }
              }
            }
            frame "L" {
              # "waypoints"
              # "headings"
              n329 = Build Array(69.0 ("element"), 126.0 ("element")) -> (w369:dbl[])
              n330 = Build Array(50.0 ("element"), 5.0 ("element")) -> (w368:dbl[])
              n331 = Array Size(array=w369) -> (size(s)=w374:i32)
              n332 = for {
                N: w374 -> [_]
                tunnel: w369 -> [w376] mode=indexing
                tunnel: w368 -> [w375] mode=indexing
                n333 = while {
                  tunnel: w376 -> [w381]
                  tunnel: w375 -> [w377]
                  stop <- w386 stop-if-true
                  # "1176.44"
                  n334 = expression code="1176.44*x"(w381) -> (w382:dbl)
                  "dis 6" <- w382
                  n335 = global read "Robot Global Data.vi" "Yaw"() -> (w378:dbl)
                  n336 = Wait (ms)(milliseconds to wait=u32 10) -> ()  [unwired: 1 out]
                  n337 = global read "Robot Global Data.vi" "Right Pos"() -> (w379:i32)
                  "Right Pos 5" <- w379
                  n338 = Subtract(x=w378, y=w377) -> (x-y=w380:dbl)
                  n339 = Greater Or Equal?(x=w379, y=w382) -> (x >= y?=w386:bool)
                  n340 = Multiply(x=w380, y="Kp 7") -> (x*y=w385:dbl)
                  n341 = Subtract(x="Speed Dr str 7", y=w385) -> (x-y=w388:dbl)
                  n342 = Add(x="Speed Dr str 7", y=w385) -> (x+y=w387:dbl)
                  n343 = global write "Robot Global Data.vi" "Auto Left Axis"(w388) -> ()
                  n344 = global write "Robot Global Data.vi" "Auto Right Axis"(w387) -> ()
                }
              }
            }
          }
        }
        frame #3 {
          w390 = 0.0 ("Intake motor")
          n345 = Wait (ms)(milliseconds to wait=u32 100) -> ()  [unwired: 1 out]
          n346 = global write "Robot Global Data.vi" "Auto Right Axis"(w390) -> ()
          n347 = global write "Robot Global Data.vi" "Auto Left Axis"(w390) -> ()
        }
        frame #4 {
          w393 = 0.0 ("Auto Right Axis")
          n348 = Wait (ms)(milliseconds to wait=u32 100) -> ()  [unwired: 1 out]
          n349 = global write "Robot Global Data.vi" "Auto Right Axis"(w393) -> ()
          n350 = global write "Robot Global Data.vi" "Auto Left Axis"(w393) -> ()
        }
        frame #5 {
          n351 = Tick Count (ms)() -> (millisecond timer value=w394:u32)
          n352 = while {
            tunnel: w394 -> [w399]
            stop <- w396 stop-if-true
            n353 = Tick Count (ms)() -> (millisecond timer value=w400:u32)
            n354 = global write "Robot Global Data.vi" "Intake motor"(-1.0 ("Intake motor")) -> ()
            n355 = Wait (ms)(milliseconds to wait=u32 10) -> ()  [unwired: 1 out]
            n356 = Subtract(x=w400, y=w399) -> (x-y=w398:u32)
            n357 = Greater?(x=w398, y=u32 700) -> (0:w396:bool)
          }
        }
        frame #6 {
          n358 = global write "Robot Global Data.vi" "Intake motor"(0.0 ("Intake motor")) -> ()
          n359 = Wait (ms)(milliseconds to wait=u32 500) -> ()  [unwired: 1 out]
        }
      }
    }
    frame 5 {
      n360 = flat-sequence {
        frame #0 {
        }
      }
    }
  }
